vi "Max and Min Location.vi"(0 "Array":dbl[][](array[numeric]), 5 "x multiplier":dbl, 7 "x offset":dbl, 9 "y multiplier":dbl, 11 "y offset":dbl) -> (4 "max value":dbl, 6 "Fast Axis Pos (Max)":dbl, 8 "Slow Axis Pos (Max)":dbl, 10 "min value":dbl)   [LabVIEW 2021]
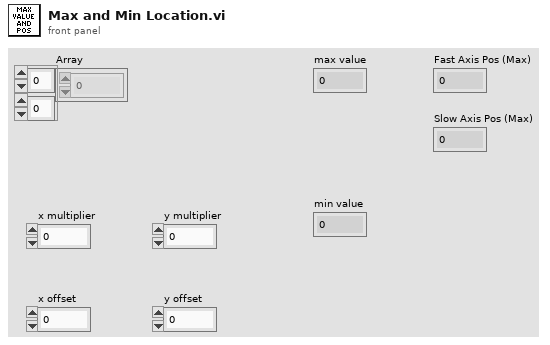
[diagram p1: front panel]
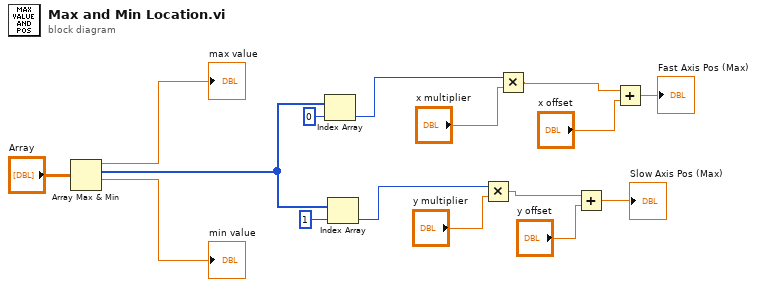
[diagram p0: block diagram]
diagram:
  n1 = Array Max & Min(array="Array") -> (max value=→"max value":dbl, max index (indices)=w4:i32[], min value=→"min value":dbl)  [unwired: 1 out]
  n2 = Index Array(array=w4, index=0) -> (element=w6:i32)
  n3 = Index Array(array=w4, index=1) -> (element=w2:i32)
  n4 = Multiply(x=w2, y="y multiplier") -> (x*y=w9:dbl)
  n5 = Multiply(x=w6, y="x multiplier") -> (x*y=w12:dbl)
  n6 = Add(x=w9, y="y offset") -> (x+y=→"Slow Axis Pos (Max)":dbl)
  n7 = Add(x=w12, y="x offset") -> (x+y=→"Fast Axis Pos (Max)":dbl)
